vi "3D Cartesian Coordinate Rotation (Euler) (Scalar).vi"(6 "rotation order":T1=10 items=["X-Y-Z", "X-Z-Y", "Y-X-Z", "Y-Z-X", "Z-X-Y", "Z-Y-X", "X-Y-X", "X-Z-X", "Y-X-Y", "Y-Z-Y", "Z-X-Z", "Z-Y-Z"], 8 "Euler Angles":cluster{"phi":dbl, "theta":dbl, "psi":dbl}, 9 "z":dbl, 10 "y":dbl, 11 "x":dbl) -> (0 "error":i32, 1 "z out":dbl, 2 "y out":dbl, 3 "x out":dbl)   [LabVIEW 2020, in "NI_AALPro.lvlib"]
doc: "Rotates a three-dimensional Cartesian coordinate system in the counterclockwise direction using the Euler angles method and returns the new coordinate of the given point. Wire data to the <B>X</B> input to determine the polymorphic instance to use or manually select the instance."
uses:
  <vilib>/Analysis/NI_AALPro.lvlib
  <vilib>/Analysis/coordinate.llb/Euler Rotation Order.ctl
  <resource>/lvanlys.dll
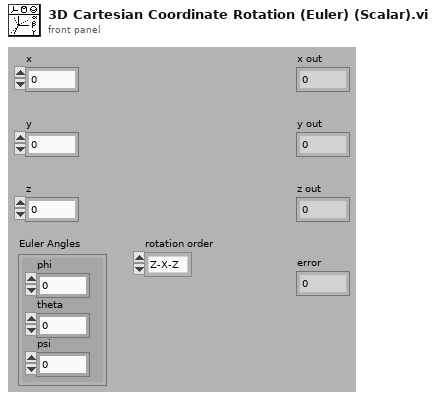
[diagram p1: front panel]
types:
  T1 = typedef "NI_AALPro.lvlib/Euler Rotation Order.ctl" = u16
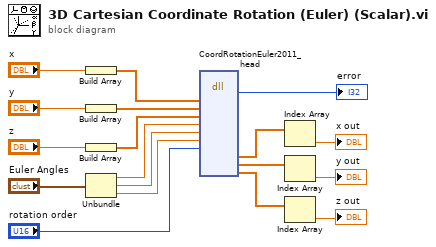
[diagram p0: block diagram]
diagram:
  n1 = Build Array("x") -> (w14:dbl[])
  n2 = Build Array("y") -> (w13:dbl[])
  n3 = Build Array("z") -> (w12:dbl[])
  n4 = Unbundle("Euler Angles") -> ("phi"=w9:dbl, "theta"=w8:dbl, "psi"=w7:dbl)
  n5 = dll-call lib="e:/builds/penguin/labview/branches/2020/dev/dist/resource/lvanlys.*" fn="CoordRotationEuler2011_head"("X"=w14, "Y"=w13, "Z"=w12, "phi"=w9, "theta"=w8, "psi"=w7, "rotateOrder"="rotation order") -> ("return type"=→"error":i32, "Xout"=w6:dbl[], "Yout"=w5:dbl[], "Zout"=w4:dbl[])  [unwired: 13 in, 2 out]
  n6 = Index Array(array=w6) -> (element=→"x out":dbl)  [unwired: 1 in]
  n7 = Index Array(array=w5) -> (element=→"y out":dbl)  [unwired: 1 in]
  n8 = Index Array(array=w4) -> (element=→"z out":dbl)  [unwired: 1 in]
